vi "Inches to Encorder Ticks.vi"(2 "distance(inches)":dbl) -> (0 "encoder distance":dbl)   [LabVIEW 2014]
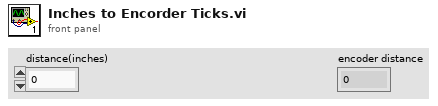
[diagram p1: front panel]
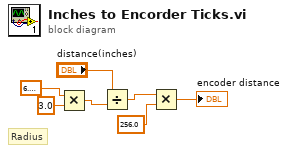
[diagram p0: block diagram]
diagram:
  # "Radius"
  n1 = Multiply(x=6.283185307179586, y=3.0) -> (x*y=w5:dbl)
  n2 = Divide(x="distance(inches)", y=w5) -> (x/y=w3:dbl)
  n3 = Multiply(x=w3, y=256.0) -> (x*y=→"encoder distance":dbl)
